vi "StateMachineProgram1MarcoGonzalez.vi"() -> ()   [LabVIEW 2012]
doc: "This VI utilizes the state machine process through 5 phases\n1) Idle (with a 2 second delay) will go to Process 1\n2) Process 1 will give the user a choice. The choice includes: back to process 1 or onto process 3\n3) Process 2 will give the user a choice. The choice includes: onto process 3 or back to process 1\n4) Process 3 will give the user choice. The choice inlcudes: Complete or back to process 2\n\nThe font panel indicates what stage the program is currently in."
panel:
  out "String":string
  in  "Down":bool
  in  "Up":bool
  # "Marco Gonzalez\nEA3 - 6th period\n04 / 20 /2017"
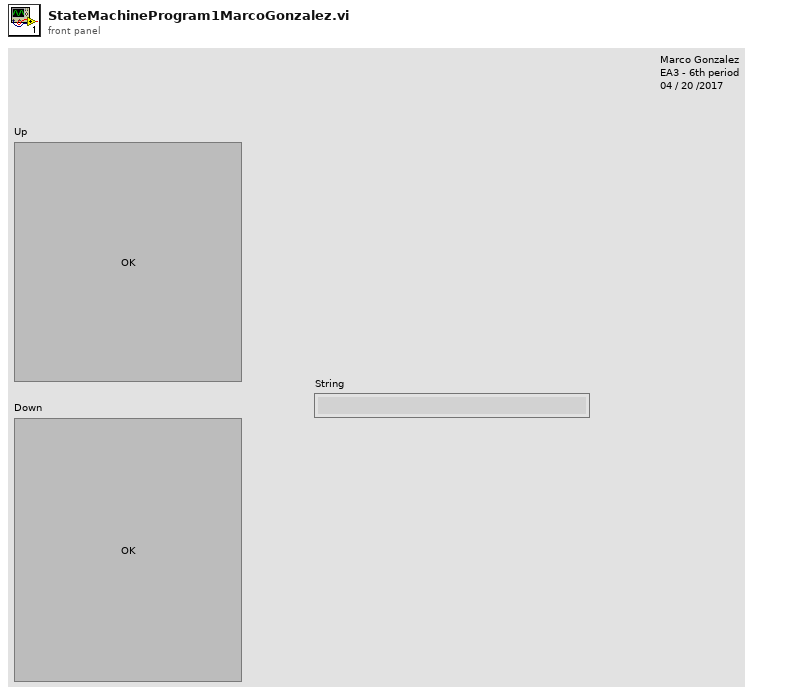
[diagram p1: front panel]
types:
  T1 = enum16{"Idle", "Process 1", "Process 2", "Process 3", "Complete"}
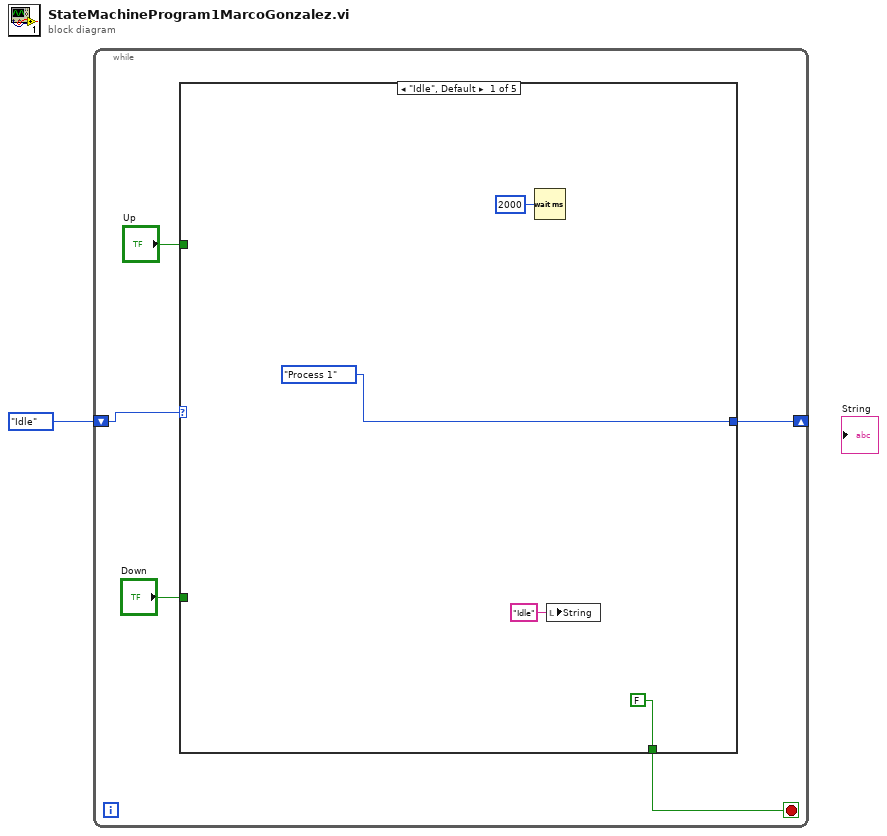
[diagram p0: block diagram]
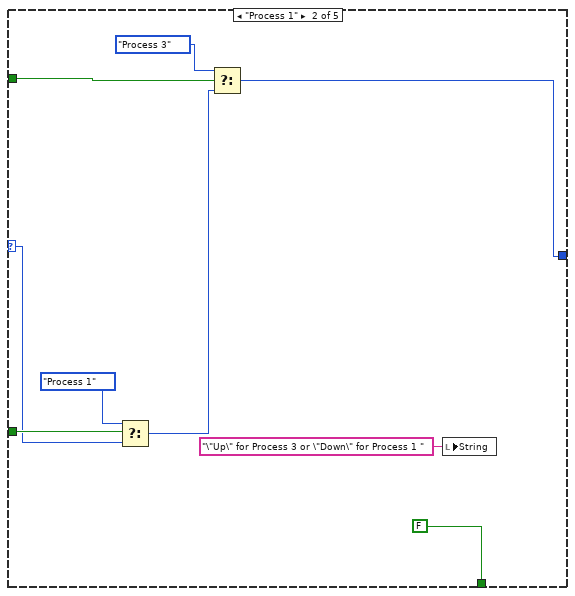
[diagram p2: hidden frame]
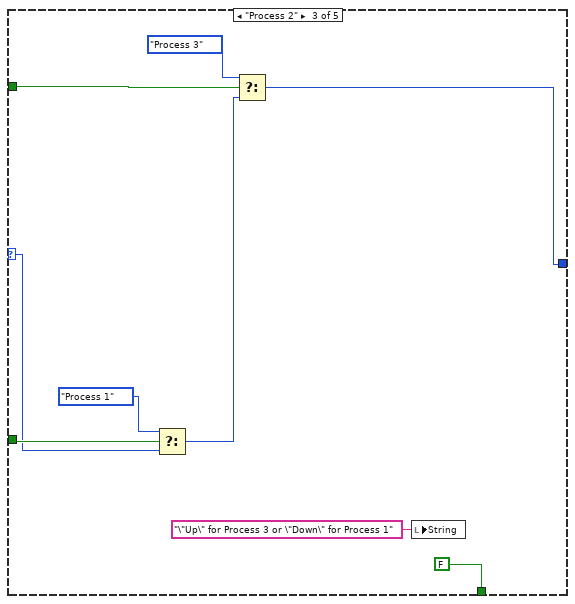
[diagram p3: hidden frame]
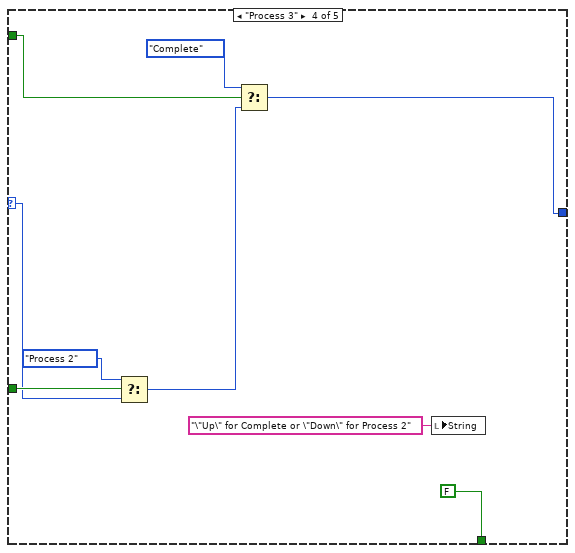
[diagram p4: hidden frame]
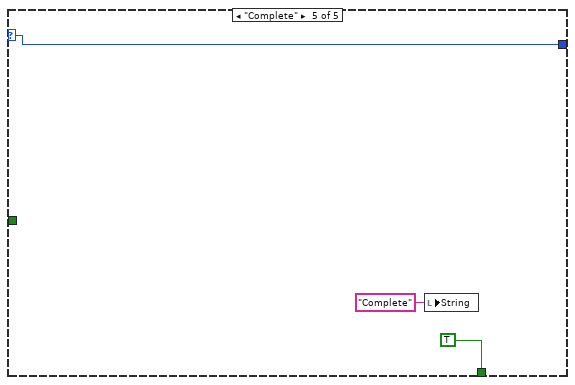
[diagram p5: hidden frame]
diagram:
  n1 = while {
    shift-right: [w2] -> _
    shift-left: T1."Idle" -> [w6]
    stop <- w3 stop-if-true
    n2 = case shown="\"Idle\", Default" w6 {
      selector: w6 -> [_ w17 w25 w36 w39]
      tunnel: "Down" -> [_ w18 w27 w37 _]
      tunnel: "Up" -> [_ w19 w28 w33 _]
      tunnel: [FALSE FALSE FALSE FALSE TRUE] -> w3
      tunnel: [T1."Process 1" ("t") w13 w21 w30 w39] -> w2
      frame "Idle", Default {
        n3 = Wait (ms)(milliseconds to wait=u32 2000) -> ()  [unwired: 1 out]
        n4 = local write "String"("Idle" ("String")) -> ()
      }
      frame "Process 1" {
        n5 = Select(t=T1."Process 1", s=w18, f=w17) -> (s? t:f=w15:T1)
        n6 = Select(t=T1."Process 3", s=w19, f=w15) -> (s? t:f=w13:T1)
        n7 = local write "String"("\"Up\" for Process 3 or \"Down\" for Process 1 " ("String")) -> ()
      }
      frame "Process 2" {
        n8 = Select(t=T1."Process 1", s=w27, f=w25) -> (s? t:f=w22:T1)
        n9 = Select(t=T1."Process 3", s=w28, f=w22) -> (s? t:f=w21:T1)
        n10 = local write "String"("\"Up\" for Process 3 or \"Down\" for Process 1" ("String")) -> ()
      }
      frame "Process 3" {
        n11 = Select(t=T1."Process 2", s=w37, f=w36) -> (s? t:f=w32:T1)
        n12 = Select(t=T1."Complete", s=w33, f=w32) -> (s? t:f=w30:T1)
        n13 = local write "String"("\"Up\" for Complete or \"Down\" for Process 2" ("String")) -> ()
      }
      frame "Complete" {
        n14 = local write "String"("Complete" ("String")) -> ()
      }
    }
  }
